vi "VannaSelection.vi"(11 "Operator Right Bumper":bool) -> ()   [LabVIEW 2019]
uses:
  Robot Global Data.vi
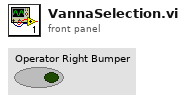
[diagram p1: front panel]
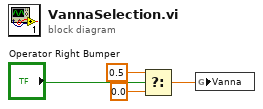
[diagram p0: block diagram]
diagram:
  n1 = Select(t=0.5, s="Operator Right Bumper", f=0.0) -> (s? t:f=w4:dbl)
  n2 = global write "Robot Global Data.vi" "Vanna"(w4) -> ()
